vi "Task Uninit.vi"(8 "error in (no error)":errorcluster, 11 "SimTask in":refnum<class "SimTask.lvclass">) -> (0 "error out":errorcluster, 3 "SimTask out":refnum<class "SimTask.lvclass">)   [LabVIEW 2020, in "VolatusDemo.lvlib" / "SimTask.lvclass"]
uses:
  SimTask.lvclass
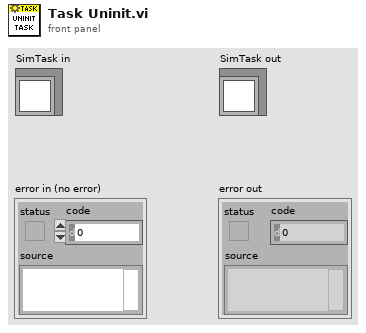
[diagram p1: front panel]
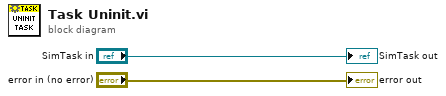
[diagram p0: block diagram]
diagram:
  "error out" <- "error in (no error)"
  "SimTask out" <- "SimTask in"
